vi "Unpack Listbox Double Click.vi"(0 "ListboxDoubleClickMsg":refnum<class "ListboxDoubleClickMsg.lvclass">) -> (3 "Listbox Label":string, 4 "Ctl Refnum":refnum<vi>, 6 "Time":u32, 8 "Coords":T2, 10 "Button":u16, 13 "Row":i32, 14 "PlatMods":T1, 15 "Mods":cluster{"Double Click":bool, "Menu Key":bool})   [LabVIEW 2015, in "ActorEvents.lvlib" / "ListboxDoubleClickMsg.lvclass"]
doc: "<License>\nCopyright © 2017 Composed Systems, LLC | All rights reserved\nwww.composed.io\n\nAuthor: Ethan Stern <ethan.stern@composed.io>\n\nThis software is provided \"AS IS\" WITHOUT WARRANTIES, either express or implied, AND IS FOR EDUCATIONAL PURPOSES ONLY.\n</License>"
uses:
  ListboxDoubleClickMsg.lvclass
  <vilib>/Utility/miscctls.llb/LVPoint32TypeDef.ctl
  ListboxDoubleClickMsg.lvclass/ListboxDoubleClickMsg.ctl
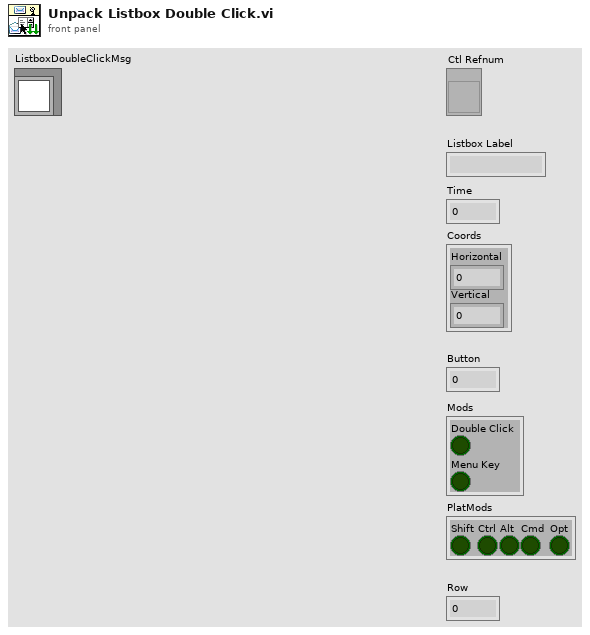
[diagram p1: front panel]
types:
  T1 = cluster{"Shift":bool, "Ctrl":bool, "Alt":bool, "Cmd":bool, "Opt":bool}
  T2 = typedef "LVPoint32TypeDef.ctl" = cluster{"Horizontal":i32, "Vertical":i32}
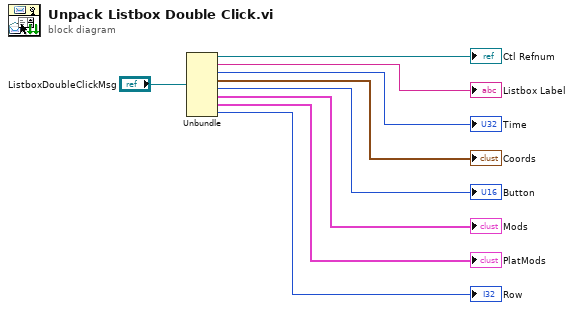
[diagram p0: block diagram]
diagram:
  n1 = Unbundle("ListboxDoubleClickMsg") -> (→"Ctl Refnum":refnum<vi>, →"Listbox Label":string, →"Time":u32, →"Coords":T2, →"Button":u16, →"Mods":cluster{"Double Click":bool, "Menu Key":bool}, →"PlatMods":T1, →"Row":i32)
